vi "Unregister.vi"(8 "error in (no error)":errorcluster, 11 "Normal Text in":refnum<class "Normal Text.lvclass">) -> (0 "error out":errorcluster, 3 "Normal Text out":refnum<class "Normal Text.lvclass">)   [LabVIEW 2011, in "Normal Text.lvclass"]
uses:
  Normal Text.lvclass
  Normal Text.lvclass/Normal Text.ctl
  Observable/Observable.lvclass
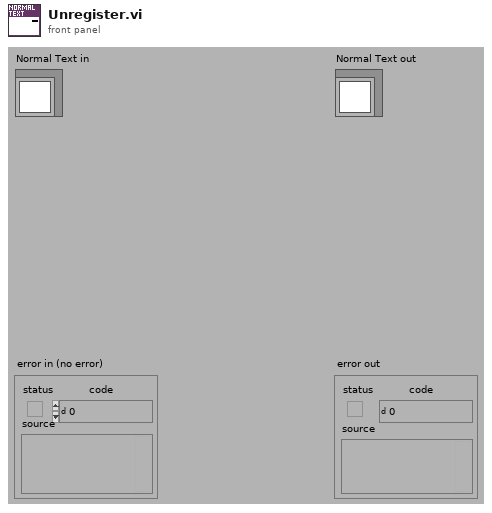
[diagram p1: front panel]
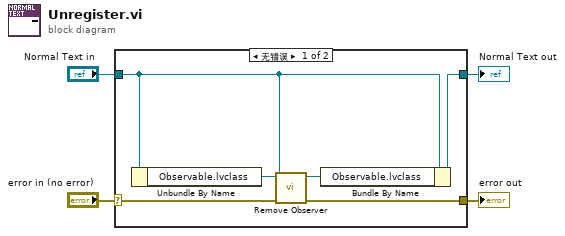
[diagram p0: block diagram]
diagram:
  n1 = case shown="无错误" "error in (no error)" {
    selector: "error in (no error)" -> [w6 w12]
    tunnel: "Normal Text in" -> [w9 w11]
    tunnel: [w7 w11] -> w3
    tunnel: [w5 w12] -> w1
    frame No Error {
      n2 = Unbundle By Name(w9) -> ("Observable.lvclass"=w10:refnum<class "Observable.lvclass">)
      n3 = call "Remove Observer.vi"("error in (no error)"=w6, "Observer"=w9, "Observable in"=w10) -> ("error out"=w5:errorcluster, "Observable out"=w8:refnum<class "Observable.lvclass">)  [unwired: 7 in]
      n4 = Bundle By Name(cluster=w9, "Observable.lvclass"=w8) -> (w7:refnum<class "Normal Text.lvclass">)
    }
    frame Error {
    }
  }
  "Normal Text out" <- w3
  "error out" <- w1
